vi "ManipEnd.vi"() -> (0 "Error Out":errorcluster, 1 "Advance Trigger":bool)   [LabVIEW 2023]
doc: "Stops the manipulator sequencer.\n\nParameters: None"
uses:
  GlobalDriverStationCommands.vi
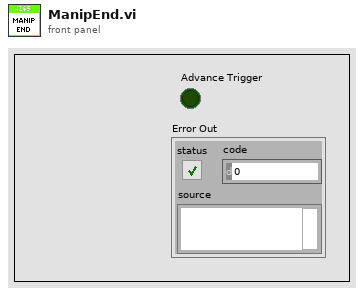
[diagram p1: front panel]
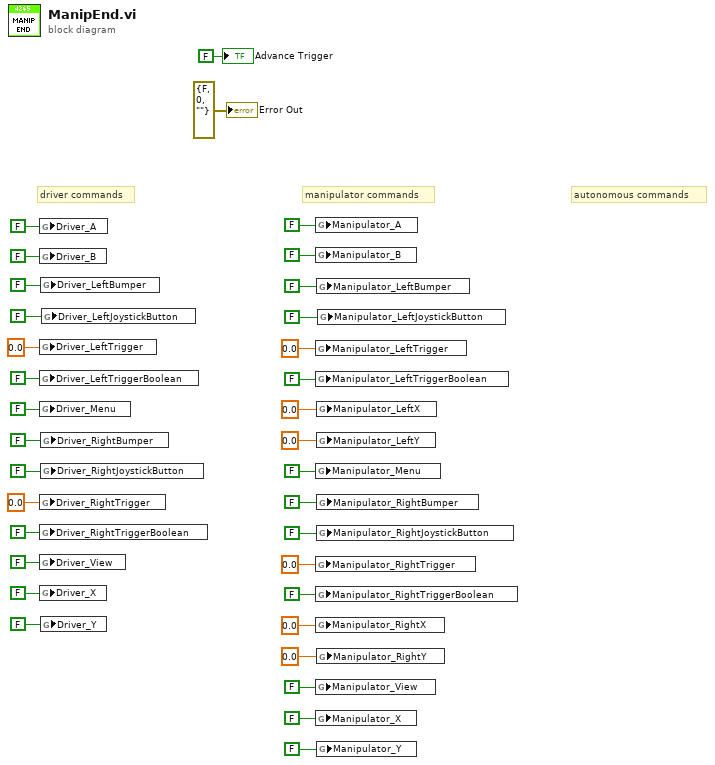
[diagram p0: block diagram]
diagram:
  # "manipulator commands"
  # "driver commands"
  # "autonomous commands"
  n1 = global write "GlobalDriverStationCommands.vi" "Driver_A"(FALSE ("Driver_A")) -> ()
  n2 = global write "GlobalDriverStationCommands.vi" "Driver_B"(FALSE ("Driver_B")) -> ()
  n3 = global write "GlobalDriverStationCommands.vi" "Driver_LeftTrigger"(0.0 ("Driver_LeftTrigger")) -> ()
  n4 = global write "GlobalDriverStationCommands.vi" "Driver_LeftTriggerBoolean"(FALSE ("Driver_LeftTriggerBoolean")) -> ()
  n5 = global write "GlobalDriverStationCommands.vi" "Driver_Menu"(FALSE ("Driver_Menu")) -> ()
  n6 = global write "GlobalDriverStationCommands.vi" "Driver_RightTrigger"(0.0 ("Driver_RightTrigger")) -> ()
  n7 = global write "GlobalDriverStationCommands.vi" "Driver_RightTriggerBoolean"(FALSE ("Driver_RightTriggerBoolean")) -> ()
  n8 = global write "GlobalDriverStationCommands.vi" "Driver_View"(FALSE ("Driver_View")) -> ()
  n9 = global write "GlobalDriverStationCommands.vi" "Driver_X"(FALSE ("Driver_X")) -> ()
  n10 = global write "GlobalDriverStationCommands.vi" "Driver_LeftBumper"(FALSE ("Driver_LeftBumper")) -> ()
  n11 = global write "GlobalDriverStationCommands.vi" "Driver_RightBumper"(FALSE ("Driver_RightBumper")) -> ()
  n12 = global write "GlobalDriverStationCommands.vi" "Driver_RightJoystickButton"(FALSE ("Driver_RightJoystickButton")) -> ()
  n13 = global write "GlobalDriverStationCommands.vi" "Driver_Y"(FALSE ("Driver_Y")) -> ()
  n14 = global write "GlobalDriverStationCommands.vi" "Driver_LeftJoystickButton"(FALSE ("Driver_LeftJoystickButton")) -> ()
  n15 = global write "GlobalDriverStationCommands.vi" "Manipulator_A"(FALSE ("Driver_A")) -> ()
  n16 = global write "GlobalDriverStationCommands.vi" "Manipulator_B"(FALSE ("Driver_B")) -> ()
  n17 = global write "GlobalDriverStationCommands.vi" "Manipulator_LeftTrigger"(0.0 ("Driver_LeftTrigger")) -> ()
  n18 = global write "GlobalDriverStationCommands.vi" "Manipulator_LeftTriggerBoolean"(FALSE ("Driver_LeftTriggerBoolean")) -> ()
  n19 = global write "GlobalDriverStationCommands.vi" "Manipulator_Menu"(FALSE ("Driver_Menu")) -> ()
  n20 = global write "GlobalDriverStationCommands.vi" "Manipulator_RightTrigger"(0.0 ("Driver_RightTrigger")) -> ()
  n21 = global write "GlobalDriverStationCommands.vi" "Manipulator_RightTriggerBoolean"(FALSE ("Driver_RightTriggerBoolean")) -> ()
  n22 = global write "GlobalDriverStationCommands.vi" "Manipulator_RightX"(0.0 ("Driver_RightX")) -> ()
  n23 = global write "GlobalDriverStationCommands.vi" "Manipulator_View"(FALSE ("Driver_View")) -> ()
  n24 = global write "GlobalDriverStationCommands.vi" "Manipulator_X"(FALSE ("Driver_X")) -> ()
  n25 = global write "GlobalDriverStationCommands.vi" "Manipulator_LeftBumper"(FALSE ("Driver_LeftBumper")) -> ()
  n26 = global write "GlobalDriverStationCommands.vi" "Manipulator_LeftX"(0.0 ("Driver_LeftX")) -> ()
  n27 = global write "GlobalDriverStationCommands.vi" "Manipulator_LeftY"(0.0 ("Driver_LeftY")) -> ()
  n28 = global write "GlobalDriverStationCommands.vi" "Manipulator_RightBumper"(FALSE ("Driver_RightBumper")) -> ()
  n29 = global write "GlobalDriverStationCommands.vi" "Manipulator_RightJoystickButton"(FALSE ("Driver_RightJoystickButton")) -> ()
  n30 = global write "GlobalDriverStationCommands.vi" "Manipulator_RightY"(0.0 ("Driver_RightY")) -> ()
  n31 = global write "GlobalDriverStationCommands.vi" "Manipulator_Y"(FALSE ("Driver_Y")) -> ()
  n32 = global write "GlobalDriverStationCommands.vi" "Manipulator_LeftJoystickButton"(FALSE ("Driver_LeftJoystickButton")) -> ()
  "Advance Trigger" <- FALSE ("Advance Trigger")
  "Error Out" <- errorcluster {"status"=FALSE, "code"=0, "source"=""} ("error constant")
